vi "Insert table.vi"() -> ()   [LabVIEW 2015]
uses:
  <vilib>/addons/database/Connection.llb/DB Tools Open Connec (Path).vi
  <vilib>/addons/database/Connection.llb/Conn Execute.vi
  <vilib>/addons/database/Recordset.llb/Rec Destroy - Connection.vi
  <vilib>/addons/database/NI_Database_API.lvlib
panel:
  in  "dbn":dbl format="%#_13g"
  in  "Number":i32
  in  "Name":string
  in  "connection information":path
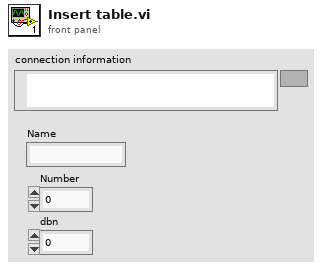
[diagram p1: front panel]
types:
  T1 = typedef "NI_Database_API.lvlib/Conn ObjectReference.ctl" = refnum<k1>
  T2 = typedef "NI_Database_API.lvlib/Rec ObjectReference.ctl" = refnum<k1>
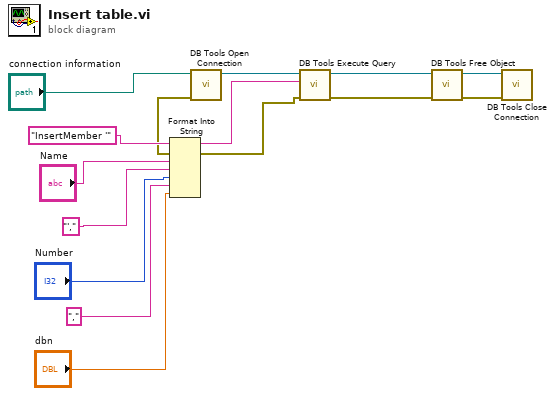
[diagram p0: block diagram]
diagram:
  n1 = call-poly <vilib>:"DB Tools Open Connection.vi"("connection information"="connection information") -> ("error out"=w8:errorcluster, "connection reference"=w12:T1)  [unwired: 7 in]
  n2 = Format Into String(initial string="InsertMember '" ("SQL query"), error in=w8, "Name", "',", "Number", ",", "dbn") -> (resulting string=w11:string, error out=w9:errorcluster)  [unwired: 1 in]
  n3 = call-poly <vilib>:"DB Tools Execute Query.vi"("error in (no error)"=w9, "SQL query"=w11, "connection reference"=w12) -> ("error out"=w1:errorcluster, "recordset reference"=w2:T2)  [unwired: 5 in]
  n4 = call-poly <vilib>:"DB Tools Free Object.vi"("error in (no error)"=w1, "recordset reference"=w2) -> ("error out"=w15:errorcluster, "connection reference"=w14:T1)  [unwired: 8 in]
  n5 = call <vilib>:"DB Tools Close Connection.vi"("error in (no error)"=w15, "connection reference"=w14) -> ()  [unwired: 5 in, 1 out]
